vi "Write Register.vi"(0 "RS485 reference":refnum<class "Modbus Master.lvclass">, 1 "Value to write":u16, 2 "Starting address":u16, 3 "Serial reference":refnum<visa-resource-name>, 4 "Serial?":bool, 5 "error in":errorcluster) -> (14 "RS485 out":refnum<class "Modbus Master.lvclass">, 17 "Serial reference out":refnum<visa-resource-name>, 19 "error out":errorcluster)   [LabVIEW 2023]
uses:
  <vilib>/NI/Modbus Library/API/Master/Modbus Master.lvclass
  RS485/RS485.lvlib
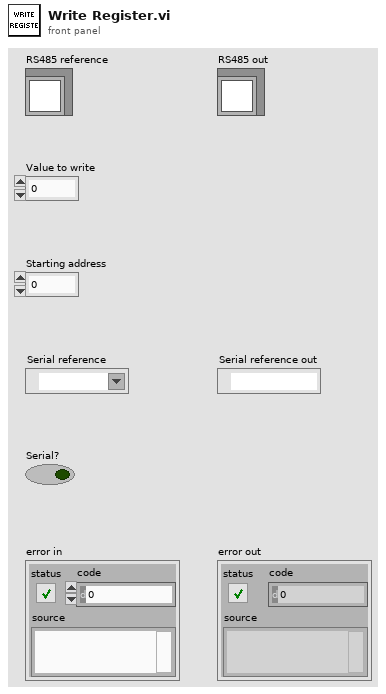
[diagram p1: front panel]
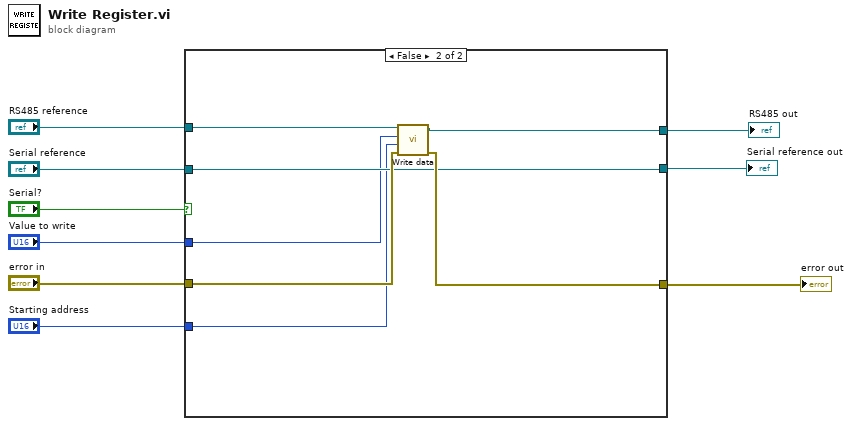
[diagram p0: block diagram]
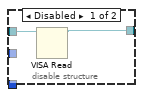
[diagram p3: hidden frame]
diagram:
  n1 = case shown="False" "Serial?" {
    tunnel: "RS485 reference" -> [w14 w25]
    tunnel: "Serial reference" -> [w15 w21]
    tunnel: "error in" -> [w12 w24]
    tunnel: "Value to write" -> [w11 w19]
    tunnel: "Starting address" -> [w10 w20]
    tunnel: [w14 w23] -> w3
    tunnel: [w12 w22] -> w2
    tunnel: [w13 w21] -> w1
    frame True {
      n2 = disable-structure shown="Enabled" {
        disable-tunnel: w15 -> [w17 w18]
        disable-tunnel: [w16 w18] -> w13
        disable-tunnel: w11 -> [_ _]
        disable-tunnel: w10 -> [_ _]
        frame Disabled {
          n3 = VISA Read(VISA resource name=w17) -> (VISA resource name out=w16:refnum<visa-resource-name>)  [unwired: 2 in, 3 out]
        }
        frame Enabled {
        }
      }
    }
    frame False {
      n4 = call "Write data.vi"("error in"=w24, "starting address"=w20, "register to write"=w19, "Modbus master in"=w25) -> ("error out"=w22:errorcluster, "Modbus master out"=w23:refnum<class "Modbus Master.lvclass">)  [unwired: 6 in]
    }
  }
  "RS485 out" <- w3
  "error out" <- w2
  "Serial reference out" <- w1
